vi "Read configuration.vi"(8 "error in":errorcluster, 11 "tag bus configurable plugin editor node in":refnum<class "user control module editor.lvclass">) -> (0 "error out":errorcluster, 2 "configuration":refnum<class "NISE_CEF_serializable configuration.lvclass">, 3 "tag bus configurable plugin editor node out":refnum<class "user control module editor.lvclass">)   [LabVIEW 2013, in "user control module editor.lvclass"]
uses:
  user control module editor.lvclass
  <vilib>/NI/Configuration Framework/serializable configuration/NISE_CEF_serializable configuration.lvclass
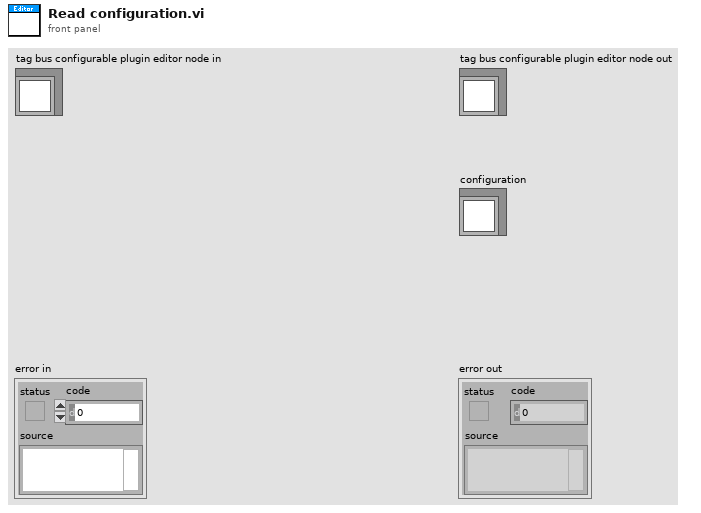
[diagram p1: front panel]
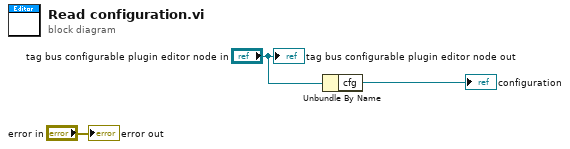
[diagram p0: block diagram]
diagram:
  n1 = Unbundle By Name("tag bus configurable plugin editor node in") -> ("cfg"=→"configuration":refnum<class "user control module configuration.lvclass">)
  "error out" <- "error in"
  "tag bus configurable plugin editor node out" <- "tag bus configurable plugin editor node in"
